vi "Data_GetFilePath.vi"(8 "error in (no error)":errorcluster, 11 "data":variant) -> (0 "error out":errorcluster, 3 "path":path)   [LabVIEW 2017, in "FileManager.lvlib"]
uses:
  <vilib>/addons/InsightCM/Devices/Shared/Common/FileManager/FileManager.lvlib
  <vilib>/addons/InsightCM/Devices/Shared/Common/FileManager/controls/DataPropertyNames.ctl
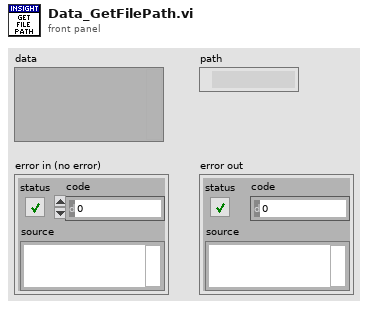
[diagram p1: front panel]
types:
  T1 = typedef "DataPropertyNames.ctl" = enum16{"Type", "EventRef", "FilePath", "DataGroup", "AcquisitionTimestamp", "StreamId", "StreamBlock", "TrendPointsOnly", "ExtraLargeFile"}
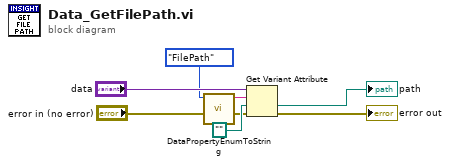
[diagram p0: block diagram]
diagram:
  n1 = call <vilib>:"DataPropertyEnumToString.vi"("property"=DataPropertyNames."FilePath" ("Names")) -> ("string"=w1:string)  [unwired: 10 in]
  n2 = Get Variant Attribute(Variant="data", name=w1, default value (empty Variant)=path "", error in="error in (no error)") -> (value=→"path":path, error out=→"error out":errorcluster)  [unwired: 2 out]
